vi "parseFunction.vi"(8 "error in (no error)":errorcluster, 11 "FrameParser in":refnum<class "FrameParser.lvclass">) -> (0 "error out":errorcluster, 2 "Function":u8, 3 "FrameParser out":refnum<class "FrameParser.lvclass">)   [LabVIEW 2015, in "RTModbus.lvlib" / "FrameParser.lvclass"]
uses:
  FrameParser.lvclass
  FrameParser.lvclass/FrameParser.ctl
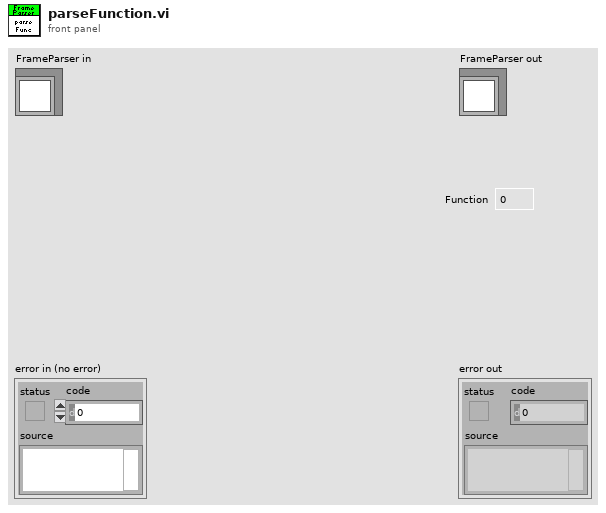
[diagram p1: front panel]
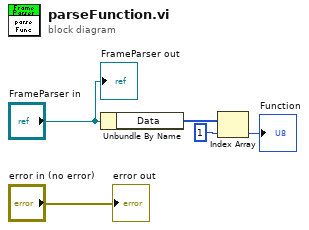
[diagram p0: block diagram]
diagram:
  n1 = Unbundle By Name("FrameParser in") -> ("Data"=w5:u8[])
  n2 = Index Array(array=w5, index=1) -> (element=→"Function":u8)
  "error out" <- "error in (no error)"
  "FrameParser out" <- "FrameParser in"
